vi "Get Oscillator Frequency.vi"(11 "Array 3":string[](array[string])) -> (1 "Oscillator Freqs":dbl[](array[numeric]), 3 "Tuning Word":string[](array[string]))   [LabVIEW 2018]
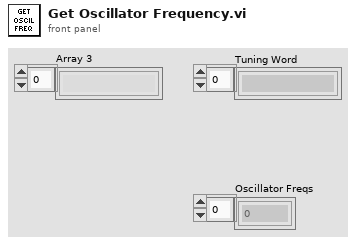
[diagram p1: front panel]
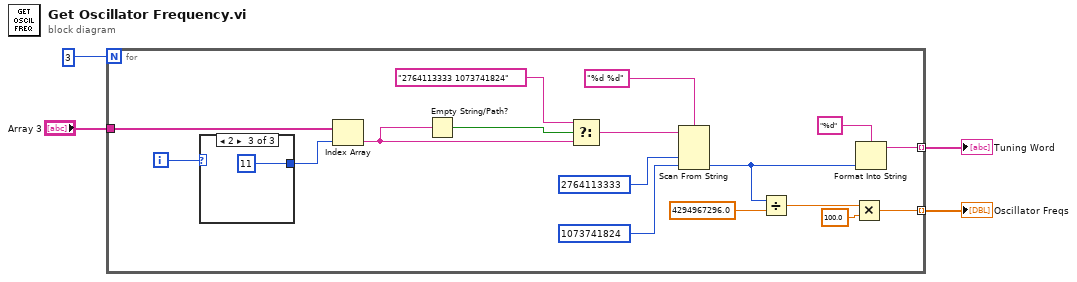
[diagram p0: block diagram]
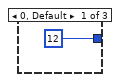
[diagram p2: hidden frame]
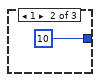
[diagram p3: hidden frame]
diagram:
  n1 = for {
    N: 3 -> [_]
    tunnel: "Array 3" -> [w20]
    tunnel: [w8] -> w4 mode=indexing
    tunnel: [w5] -> w3 mode=indexing
    i -> [w21]
    n2 = case shown="2" w21 {
      tunnel: [12 ("y") 10 ("y") 11 ("y")] -> w19
      frame 0, Default {
      }
      frame 1 {
      }
      frame 2 {
      }
    }
    n3 = Index Array(array=w20, index=w19) -> (element=w14:string)
    n4 = Empty String/Path?(string/path=w14) -> (empty?=w17:bool)
    n5 = Select(t="2764113333 1073741824", s=w17, f=w14) -> (s? t:f=w15:string)
    n6 = Scan From String(format string="%d %d", input string=w15, default 1=u32 2764113333 ("default value 1"), default 2=u32 1073741824 ("default value 1")) -> (output 2=w6:u32)  [unwired: 2 in, 4 out]
    n7 = Divide(x=w6, y=4294967296.0) -> (x/y=w10:dbl)
    n8 = Multiply(x=w10, y=100.0) -> (x*y=w8:dbl)
    n9 = Format Into String(format string="%d", w6) -> (resulting string=w5:string)  [unwired: 2 in, 1 out]
  }
  "Oscillator Freqs" <- w4
  "Tuning Word" <- w3
